vi "WGC.vi"(0 "System no.":i32=1 min=1 max=4 step=1, 2 "Affected axes":string[](array[string]), 3 "Cycles":i32[](array[numeric]), 5 "error in":errorcluster) -> (14 "Controller error":bool, 19 "error out":errorcluster)   [LabVIEW 2020]
doc: "Sets number of wave generator cycles. Controller error is TRUE if selected system reports an error code which is not zero.\n\nC-413: Affected axes is identical with wave generator ID, which can be 1 to 2. If Cycles = 0 the wave is performed periodically until it is stopped otherwise. \n\nC-886: Affected axes is identical with wave generator ID, which can be 1 to No. of connected axes. If Cycles = 0 the wave is performed periodically until it is stopped otherwise. Cycles set for any wave generator ID are valid for all wave generators (cannot be set differently).\n\nC-887: Affected axes is identical with wave generator ID, which can be 1 to No. of connected axes. If Cycles = 0 the wave is performed periodically until it is stopped otherwise. Cycles set for any wave generator ID are valid for all wave generators (cannot be set differently).\n\nC-891: Affected axes is identical with wave generator ID, which can be 1. If Cycles = 0 the wave is performed periodically until it is stopped otherwise. \n\nE-517, E-518: Affected axes is identical with wave generator ID, which can be 1 to 3. If Cycles = 0 the wave is performed periodically until it is stopped otherwise. WGC saves the new value in RAM only. The WPA command saves the currently valid value to non-volatile memory, where it becomes the power-on default. Settings not saved with WPA will be lost on power down or reboot.\n\nE-709: Affected axes is identical with wave generator ID, which can be 1. If Cycles = 0 the wave is performed periodically until it is stopped otherwise.\n\nE-712: Affected axes is identical with wave generator ID, which can be 1 to No. of connected axes. If Cycles = 0 the wave is performed periodically until it is stopped otherwise. Cycles set for any wave generator ID are valid for all wave generators (cannot be set differently).\n\nE-725, E-727: Affected axes is identical with wave generator ID, which can be 1 to No. of connected axes. If Cycles = 0 the wave is performed periodically until it is stopped otherwise. Cycles set for any wave generator ID are valid for all wave generators (cannot be set differently).\n\nE-753: Affected axes is identical with wave generator ID, which can be 1. If Cycles = 0 the wave is performed periodically until it is stopped otherwise.\n\nE-754: Affected axes is identical with wave generator ID, which can be 1. If Cycles = 0 the wave is performed periodically until it is stopped otherwise.\n\nE-761: Affected axes is identical with wave table number, which can be 1 to 4. If Cycles = 0 the wave is performed periodically until it is stopped otherwise. E-761: WGC saves the new value in RAM only. The WPA command saves the currently valid value to non-volatile memory, where it becomes the power- on default. Settings not saved with WPA will be lost when the PC is powered off or the E-761 is rebooted."
panel:
  # "Sets number of wave generator cycles."
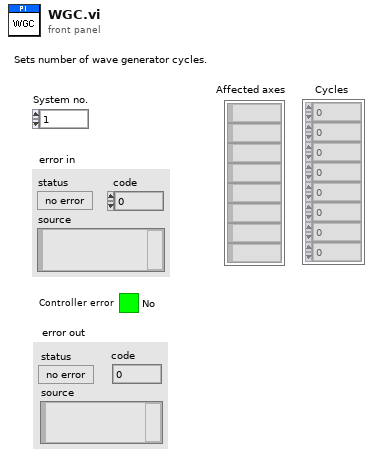
[diagram p1: front panel]
types:
  T1 = enum16{"Disable error check", "Force error check", "Use global settings"}
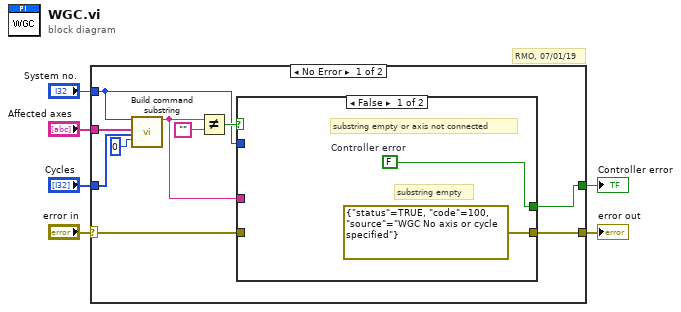
[diagram p0: block diagram]
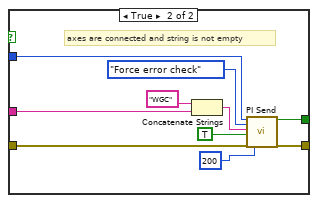
[diagram p2: hidden frame]
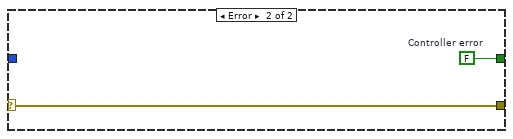
[diagram p3: hidden frame]
diagram:
  # "RMO, 07/01/19"
  n1 = case shown="No Error" "error in" {
    selector: "error in" -> [w8 w30]
    tunnel: [w16 w30] -> w6
    tunnel: "Cycles" -> [w13 _]
    tunnel: "System no." -> [w9 _]
    tunnel: "Affected axes" -> [w12 _]
    tunnel: [w7 w29] -> w1
    frame No Error {
      n2 = call "Build command substring.vi"("System no."=w9, "Affected axes"=w12, "Parameters"=w13, "No. of digits"=i16 0 ("No.of digits")) -> ("Command substring"=w14:string)  [unwired: 3 in, 12 out]
      n3 = Not Equal?(x=w14, y="") -> (x != y?=w10:bool)
      n4 = case shown="False" w10 {
        tunnel: w14 -> [_ w27]
        tunnel: [errorcluster {"status"=TRUE, "code"=100, "source"="WGC No axis or cycle specified"} ("error out") w21] -> w16
        tunnel: w8 -> [_ w24]
        tunnel: w9 -> [_ w23]
        tunnel: [w17 w20] -> w7
        frame False {
          w17 = FALSE  # Controller error
          # "substring empty"
          # "substring empty or axis not connected"
        }
        frame True {
          # "axes are connected and string is not empty"
          n5 = Concatenate Strings("WGC", w27) -> (w25:string)
          n6 = call "PI Send.vi"("System no."=w23, "Error check settings"=T1."Force error check", "String to send"=w25, "Attach termination char.?"=TRUE ("Attach Linefeed?"), "error in"=w24, "Delay before error check (ms)"=u32 200 ("milliseconds to wait")) -> ("Controller error"=w20:bool, "error out"=w21:errorcluster)  [unwired: 12 out]
        }
      }
    }
    frame Error {
      w29 = FALSE  # Controller error
    }
  }
  "error out" <- w6
  "Controller error" <- w1
